vi "Teleop_System_Acquire_Decide.vi"(11 "Teleop Elapsed Seconds":dbl) -> ()   [LabVIEW 2019]
uses:
  <vilib>/Rock Robotics/Network Tables/NT Write Numeric Array.vi
  <vilib>/Rock Robotics/Network Tables/NT Write Boolean Array.vi
  <vilib>/Rock Robotics/WPI/ThirdParty/JAS_Junk/TrajLib/Trajectory_Library.lvlib
  <vilib>/Rock Robotics/WPI/Joystick/XBox Buttons Indexer.ctl
  <vilib>/Rock Robotics/WPI/Joystick/XBox Axes Indexer.ctl
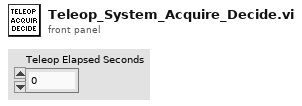
[diagram p1: front panel]
types:
  T1 = typedef "XBox Axes Indexer.ctl" = enum16{"Left X", "Left Y", "Left Trigger", "Right Trigger", "Right X", "Right Y"}
  T2 = typedef "XBox Buttons Indexer.ctl" = enum16{"A", "B", "X", "Y", "Left Bumper", "Right Bumper", "Back", "Start", "Left Joystick", "Right Joystick"}
  T3 = typedef "WPI_JoystickDevRef.ctl" = cluster{"Device":T4}
  T4 = typedef "WPI_JoystickDeviceEnum.ctl" = enum16{"USB 0", "USB 1", "USB 2", "USB 3", "USB 4", "USB 5"}
  T5 = typedef "Trajectory_Library.lvlib/TRAJ_STATE.ctl" = cluster{"TimeSeconds":dbl, "Velocity":dbl, "Acceleration":dbl, "POSE":T6, "Curvature":dbl}
  T6 = typedef "Trajectory_Library.lvlib/POSE2D.ctl" = cluster{"TRANSLATION":T7, "ROTATION":T8}
  T7 = typedef "Trajectory_Library.lvlib/TRANSLATION2D.ctl" = cluster{"X":dbl, "Y":dbl}
  T8 = typedef "Trajectory_Library.lvlib/ROTATION2D.ctl" = cluster{"VALUE":dbl, "COS":dbl, "SIN":dbl}
  T9 = cluster{"Error Pose":T6, "X Corr":dbl, "Y Corr":dbl}
  T10 = typedef "Trajectory_Library.lvlib/CHASSIS_SPEEDS.ctl" = cluster{"vX":dbl, "vY":dbl, "vOmega":dbl}
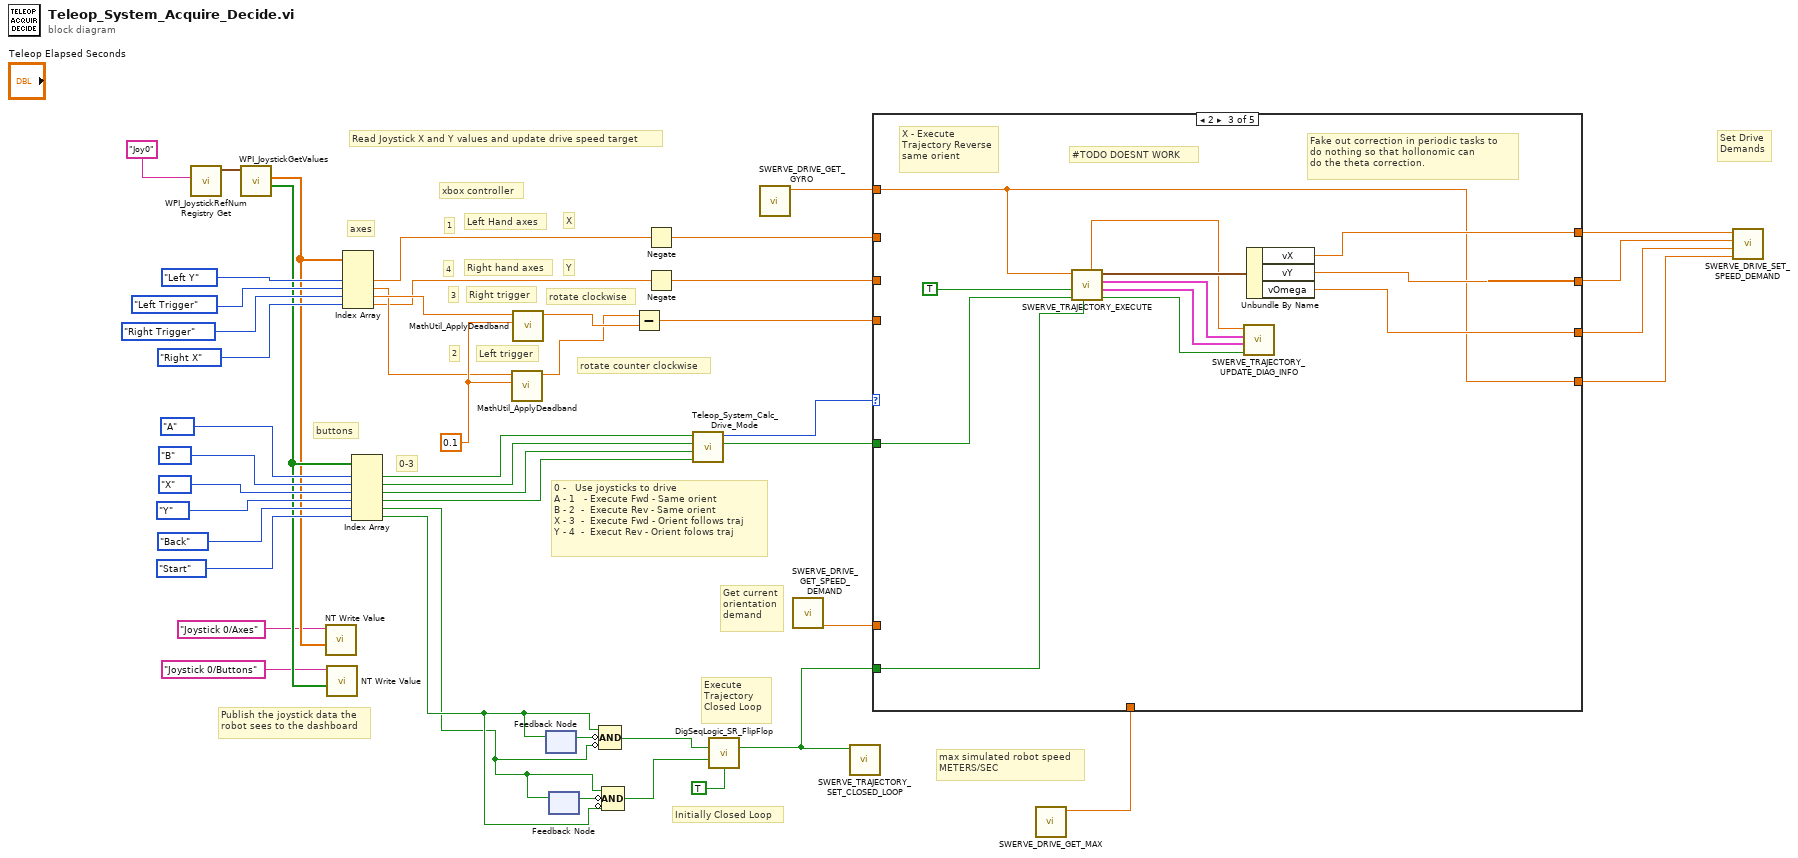
[diagram p0: block diagram]
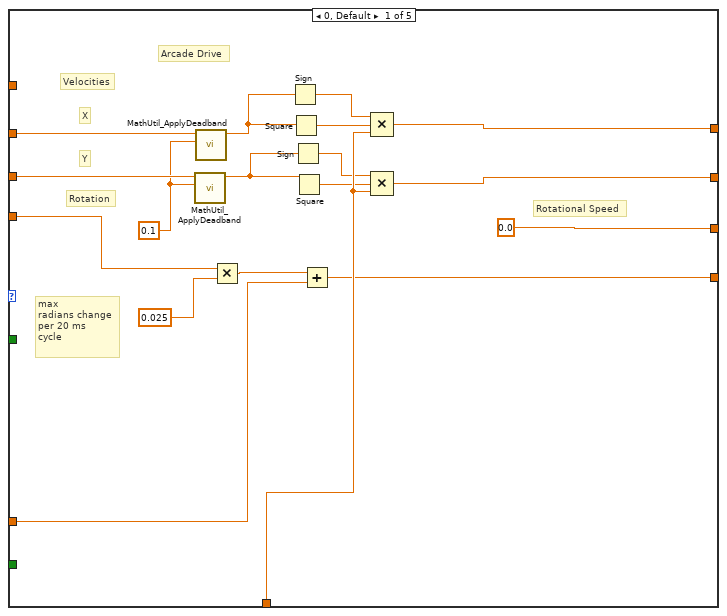
[diagram p2: hidden frame]
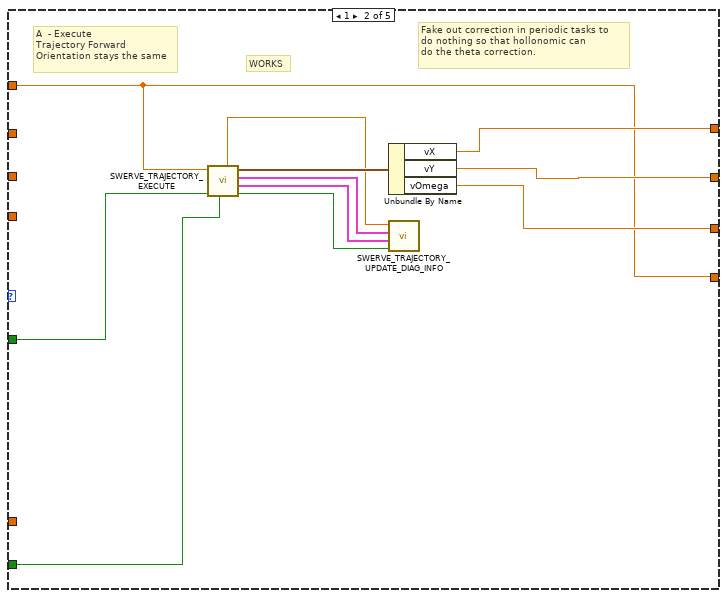
[diagram p3: hidden frame]
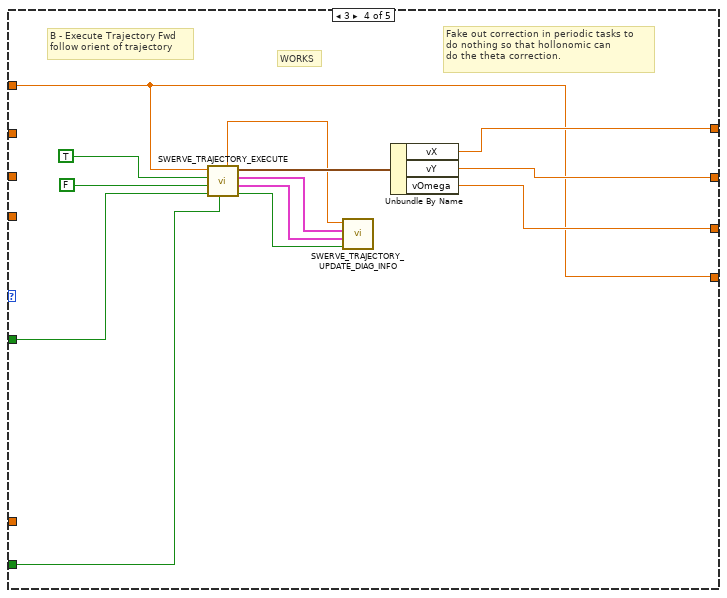
[diagram p4: hidden frame]
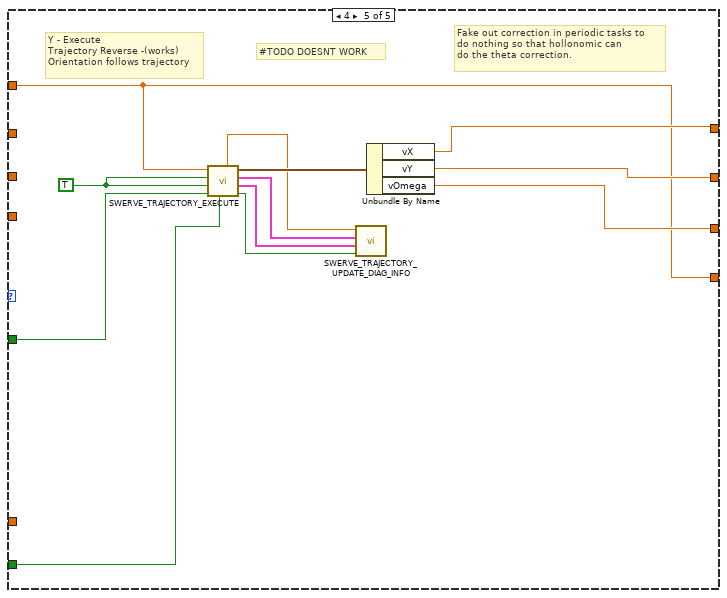
[diagram p5: hidden frame]
diagram:
  w26 = 0.1 ("Deadband")
  # "0 -   Use joysticks to drive\nA - 1   - Execute Fwd - Same orient\nB - 2  -  Execute Rev - Same orient\nX - 3  -  Execute Fwd - Orient follows traj\nY - 4  -  Execut Rev - Orient folows traj"
  # "Execute\nTrajectory\nClosed Loop"
  # "Get current\norientation\ndemand"
  # "Set Drive\nDemands"
  # "Initially Closed Loop"
  # "0-3"
  # "xbox controller"
  # "Left trigger"
  # "rotate counter clockwise"
  # "2"
  # "Right trigger"
  # "rotate clockwise"
  # "3"
  # "Left Hand axes"
  # "1"
  # "4"
  # "Right hand axes"
  # "Y"
  # "X"
  # "buttons"
  # "axes"
  # "max simulated robot speed\nMETERS/SEC"
  # "Publish the joystick data the\nrobot sees to the dashboard"
  # "Read Joystick X and Y values and update drive speed target"
  n1 = call <vilib>:"WPI_JoystickRefNum Registry Get.vi"("refnum name"="Joy0") -> ("JoystickDevRef"=w2:T3)  [unwired: 1 in, 9 out]
  n2 = call <vilib>:"WPI_JoystickGetValues.vi"("JoystickDevRef"=w2) -> ("Buttons"=w6:bool[], "Axes"=w5:dbl[])  [unwired: 6 in, 3 out]
  n3 = call-poly <vilib>:"NT Write Value.vi"("Numeric Array"=w5, "Name"="Joystick 0/Axes") -> ()  [unwired: 9 in, 1 out]
  n4 = call-poly <vilib>:"NT Write Value.vi"("Boolean Array"=w6, "Name"="Joystick 0/Buttons") -> ()  [unwired: 9 in, 1 out]
  n5 = Index Array(array=w5, index #2=XBox_Axes_Indexer."Left Y" ("XBox Axes"), index #3=XBox_Axes_Indexer."Left Trigger" ("XBox Axes"), index #4=XBox_Axes_Indexer."Right Trigger" ("XBox Axes"), index #5=XBox_Axes_Indexer."Right X" ("XBox Axes")) -> (element #2=w14:dbl, element #3=w22:dbl, element #4=w24:dbl, element #5=w15:dbl)  [unwired: 1 in, 1 out]
  n6 = Index Array(array=w6, index #1=XBox_Buttons_Indexer."A" ("XBox Buttons"), index #2=XBox_Buttons_Indexer."B" ("XBox Buttons"), index #3=XBox_Buttons_Indexer."X" ("XBox Buttons"), index #4=XBox_Buttons_Indexer."Y" ("XBox Buttons"), index #5=XBox_Buttons_Indexer."Back" ("XBox Buttons"), index #6=XBox_Buttons_Indexer."Start" ("XBox Buttons")) -> (element #1=w7:bool, element #2=w16:bool, element #3=w17:bool, element #4=w43:bool, element #5=w20:bool, element #6=w21:bool)
  n7 = call <vilib>:"MathUtil_ApplyDeadband.vi"("Deadband"=w26, "Value"=w22) -> ("Result"=w23:dbl)  [unwired: 9 in]
  n8 = call <vilib>:"MathUtil_ApplyDeadband.vi"("Deadband"=w26, "Value"=w24) -> ("Result"=w25:dbl)  [unwired: 9 in]
  n9 = feedback #1() -> (w18:bool)  [unwired: 1 in]
  n10 = feedback-in #1(w21) -> ()
  n11 = feedback #2() -> (w19:bool)  [unwired: 1 in]
  n12 = feedback-in #2(w20) -> ()
  n13 = Compound Arithmetic op=AND(w21, invert w18, invert w20) -> (w34:bool)
  n14 = Compound Arithmetic op=AND(w20, invert w19, invert w21) -> (w35:bool)
  n15 = Subtract(x=w23, y=w25) -> (x-y=w11:dbl)
  n16 = Negate(x=w14) -> (-x=w12:dbl)
  n17 = Negate(x=w15) -> (-x=w13:dbl)
  n18 = call "Teleop_System_Calc_Drive_Mode.vi"("Traj Rev Follow Orient"=w43, "Traj Rev Same Orient"=w17, "Traj Fwd Follow Orient"=w16, "Traj Fwd Same Orient"=w7) -> ("Dirve Mode Changed"=w9:bool, "Drive Mode"=w8:i32)  [unwired: 6 in]
  n19 = call <vilib>:"DigSeqLogic_SR_FlipFlop.vi"("Set"=w34, "Reset"=w35, "Initial Value"=TRUE) -> ("Output"=w36:bool)  [unwired: 11 in, 1 out]
  n20 = call "SWERVE_DRIVE_GET_GYRO.vi"() -> ("Gyro Heading Radians"=w32:dbl)  [unwired: 11 in]
  n21 = call "SWERVE_DRIVE_GET_SPEED_DEMAND.vi"() -> ("Drv Rotation Orentation Dmd"=w31:dbl)  [unwired: 8 in, 3 out]
  n22 = call "SWERVE_TRAJECTORY_SET_CLOSED_LOOP.vi"("AUTO_CLOSED_LOOP"=w36) -> ()  [unwired: 11 in]
  n23 = call "SWERVE_DRIVE_GET_MAX.vi"() -> ("Max Wheel Vel (Meter/Sec)"=w10:dbl)  [unwired: 10 in, 1 out]
  n24 = case shown="2" w8 {
    tunnel: w13 -> [w49 _ _ _ _]
    tunnel: [w65 w74 w85 w97 w110] -> w27
    tunnel: [w64 w73 w84 w96 w109] -> w28
    tunnel: w10 -> [w63 _ _ _ _]
    tunnel: w9 -> [_ w76 w88 w101 w113]
    tunnel: [w57 w70 w81 w93 w106] -> w30
    tunnel: w31 -> [w56 _ _ _ _]
    tunnel: [0.0 w72 w83 w95 w108] -> w29
    tunnel: w12 -> [w51 _ _ _ _]
    tunnel: w11 -> [w53 _ _ _ _]
    tunnel: w32 -> [_ w70 w81 w93 w106]
    tunnel: w36 -> [_ w71 w82 w94 w107]
    frame 0, Default {
      w48 = 0.1 ("Deadband")
      # "Velocities"
      # "Rotation"
      # "Rotational Speed"
      # "max \nradians change\nper 20 ms\ncycle"
      # "Y"
      # "X"
      # "Arcade Drive"
      n25 = call <vilib>:"MathUtil_ApplyDeadband.vi"("Deadband"=w48, "Value"=w49) -> ("Result"=w52:dbl)  [unwired: 9 in]
      n26 = call <vilib>:"MathUtil_ApplyDeadband.vi"("Deadband"=w48, "Value"=w51) -> ("Result"=w50:dbl)  [unwired: 9 in]
      n27 = Multiply(x=w53, y=0.025) -> (x*y=w55:dbl)
      n28 = Sign(1:w50) -> (0:w61:dbl)
      n29 = Square(x=w50) -> (x^2=w62:dbl)
      n30 = Sign(1:w52) -> (0:w59:dbl)
      n31 = Square(x=w52) -> (x^2=w60:dbl)
      n32 = Add(x=w55, y=w56) -> (x+y=w57:dbl)
      n33 = Compound Arithmetic op=MULTIPLY(w61, w62, w63) -> (w65:dbl)
      n34 = Compound Arithmetic op=MULTIPLY(w59, w60, w63) -> (w64:dbl)
    }
    frame 1 {
      # "Fake out correction in periodic tasks to \ndo nothing so that hollonomic can\ndo the theta correction."
      # "WORKS"
      # "A  - Execute\nTrajectory Forward\nOrientation stays the same"
      n35 = call "SWERVE_TRAJECTORY_EXECUTE.vi"("EnableClosedLoop"=w71, "Init"=w76, "Gyro Heading\nRAD"=w70) -> ("AtReference"=w66:bool, "OutputTRAJ_STATE"=w67:T5, "Error and Corr"=w68:T9, "Chassis Velocity Target"=w75:T10, "Orientation Target"=w69:dbl)  [unwired: 4 in]
      n36 = Unbundle By Name(w75) -> ("vX"=w74:dbl, "vY"=w73:dbl, "vOmega"=w72:dbl)
      n37 = call "SWERVE_TRAJECTORY_UPDATE_DIAG_INFO.vi"("AtReference"=w66, "OutputTRAJ_STATE"=w67, "Error and Corr"=w68, "Orientation Target"=w69) -> ()  [unwired: 8 in]
    }
    frame 2 {
      # "Fake out correction in periodic tasks to \ndo nothing so that hollonomic can\ndo the theta correction."
      # "#TODO DOESNT WORK"
      # "X - Execute \nTrajectory Reverse\nsame orient"
      n38 = call "SWERVE_TRAJECTORY_EXECUTE.vi"("EnableClosedLoop"=w82, "Init"=w88, "Reverse"=TRUE, "Gyro Heading\nRAD"=w81) -> ("AtReference"=w77:bool, "OutputTRAJ_STATE"=w78:T5, "Error and Corr"=w79:T9, "Chassis Velocity Target"=w86:T10, "Orientation Target"=w80:dbl)  [unwired: 3 in]
      n39 = call "SWERVE_TRAJECTORY_UPDATE_DIAG_INFO.vi"("AtReference"=w77, "OutputTRAJ_STATE"=w78, "Error and Corr"=w79, "Orientation Target"=w80) -> ()  [unwired: 8 in]
      n40 = Unbundle By Name(w86) -> ("vX"=w85:dbl, "vY"=w84:dbl, "vOmega"=w83:dbl)
    }
    frame 3 {
      # "Fake out correction in periodic tasks to \ndo nothing so that hollonomic can\ndo the theta correction."
      # "WORKS"
      # "B - Execute Trajectory Fwd \nfollow orient of trajectory"
      n41 = call "SWERVE_TRAJECTORY_EXECUTE.vi"("EnableClosedLoop"=w94, "Init"=w101, "Reverse"=FALSE, "Follow Orientation"=TRUE ("Reverse"), "Gyro Heading\nRAD"=w93) -> ("AtReference"=w89:bool, "OutputTRAJ_STATE"=w90:T5, "Error and Corr"=w91:T9, "Chassis Velocity Target"=w98:T10, "Orientation Target"=w92:dbl)  [unwired: 2 in]
      n42 = call "SWERVE_TRAJECTORY_UPDATE_DIAG_INFO.vi"("AtReference"=w89, "OutputTRAJ_STATE"=w90, "Error and Corr"=w91, "Orientation Target"=w92) -> ()  [unwired: 8 in]
      n43 = Unbundle By Name(w98) -> ("vX"=w97:dbl, "vY"=w96:dbl, "vOmega"=w95:dbl)
    }
    frame 4 {
      w112 = TRUE ("Reverse")
      # "Fake out correction in periodic tasks to \ndo nothing so that hollonomic can\ndo the theta correction."
      # "#TODO DOESNT WORK"
      # "Y - Execute\nTrajectory Reverse -(works)\nOrientation follows trajectory"
      n44 = call "SWERVE_TRAJECTORY_EXECUTE.vi"("EnableClosedLoop"=w107, "Init"=w113, "Reverse"=w112, "Follow Orientation"=w112, "Gyro Heading\nRAD"=w106) -> ("AtReference"=w102:bool, "OutputTRAJ_STATE"=w103:T5, "Error and Corr"=w104:T9, "Chassis Velocity Target"=w111:T10, "Orientation Target"=w105:dbl)  [unwired: 2 in]
      n45 = call "SWERVE_TRAJECTORY_UPDATE_DIAG_INFO.vi"("AtReference"=w102, "OutputTRAJ_STATE"=w103, "Error and Corr"=w104, "Orientation Target"=w105) -> ()  [unwired: 8 in]
      n46 = Unbundle By Name(w111) -> ("vX"=w110:dbl, "vY"=w109:dbl, "vOmega"=w108:dbl)
    }
  }
  n47 = call "SWERVE_DRIVE_SET_SPEED_DEMAND.vi"("Drv Rotation Orentation Dmd"=w30, "Drv Angular Vel Dmd"=w29, "Drv Y Vel Dmd"=w28, "Drv X Vel Dmd"=w27) -> ()  [unwired: 8 in]
